vi "读取信息.vi"() -> (1 "String":string)   [LabVIEW 2016]
panel:
  in  "cmd_std_header_t":T1
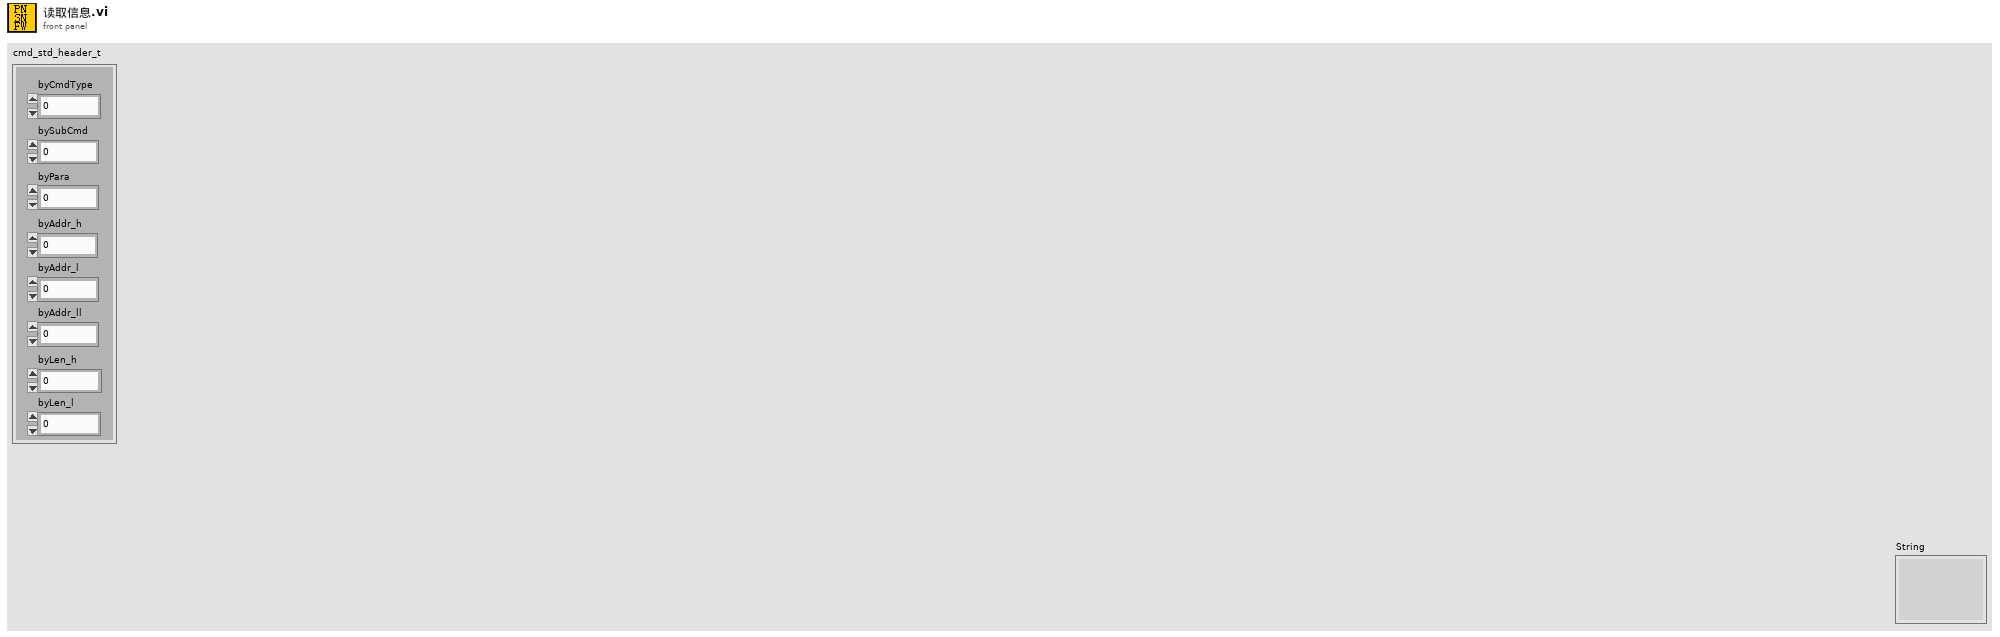
[diagram p1: front panel]
types:
  T1 = cluster{"byCmdType":u8, "bySubCmd":u8, "byPara":u8, "byAddr_h":u8, "byAddr_l":u8, "byAddr_ll":u8, "byLen_h":u8, "byLen_l":u8}
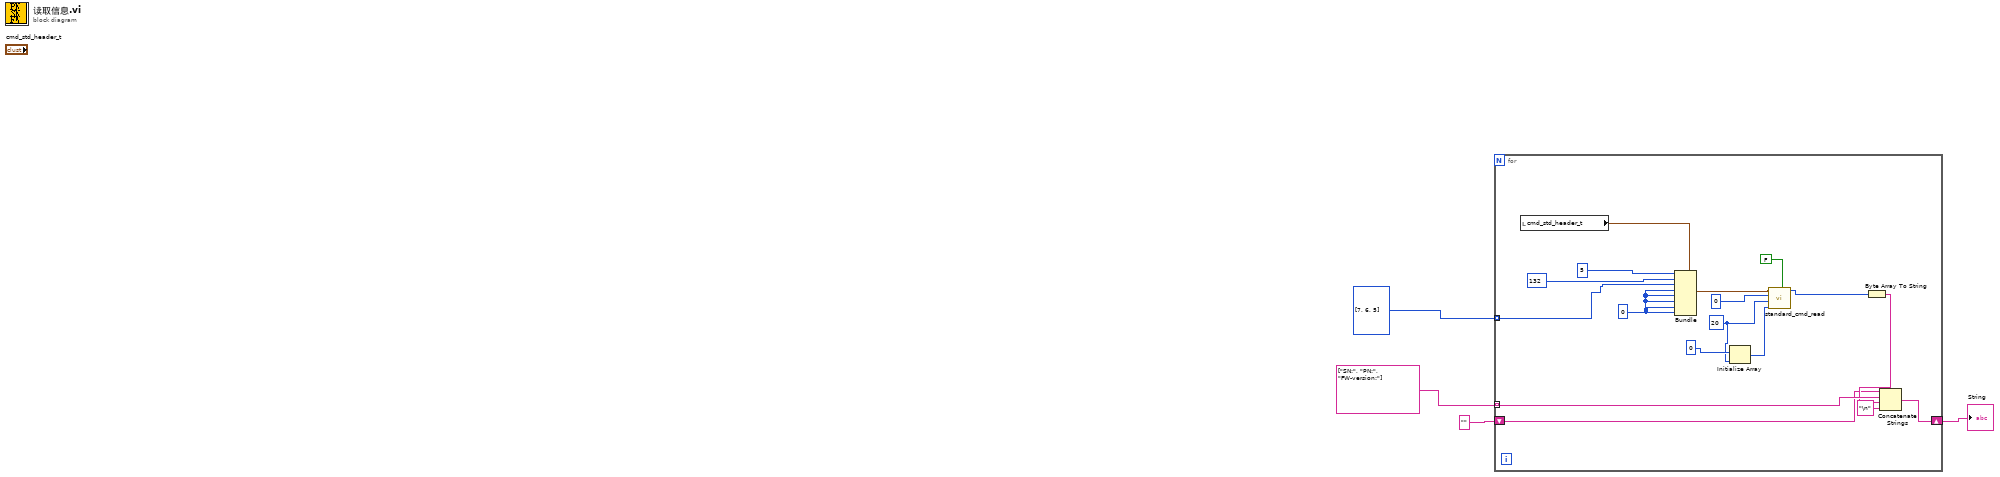
[diagram p0: block diagram]
diagram:
  n1 = for {
    tunnel: string[] ["SN:", "PN:", "FW-version:"] -> [w13] mode=indexing
    shift-right: [w10] -> w1
    shift-left: "" -> [w9]
    tunnel: u8[] [7, 6, 5] -> [w8] mode=indexing
    w5 = u32 20 ("dwLen")
    w18 = u8 0 ("byLen_l")
    n2 = local read "cmd_std_header_t"() -> (w21:T1)
    n3 = Bundle(cluster=w21, "byCmdType"=u8 5, "bySubCmd"=u8 132, "byPara"=w8, "byAddr_h"=w18, "byAddr_l"=w18, "byAddr_ll"=w18, "byLen_h"=w18, "byLen_l"=w18) -> (w17:T1)
    n4 = Initialize Array(u8 0, w5) -> (w7:u8[])
    n5 = call "standard_cmd_read.vi"("COM"=FALSE, "data"=w7, "dwLen"=w5, "dwAddr"=u32 0, "cmd_std_header_t"=w17) -> ("data out"=w15:u8[])  [unwired: 5 in, 1 out]
    n6 = Byte Array To String(unsigned byte array=w15) -> (string=w12:string)
    n7 = Concatenate Strings(w9, w13, w12, "\n" ("string")) -> (w10:string)
  }
  "String" <- w1
